vi "CHROMA Getting Started Main.vi"(8 "Error In":errorcluster) -> (0 "Error Out":errorcluster)   [LabVIEW 2016]
uses:
  Type Definition/CHROMA Voltage Range.ctl
  Type Definition/CHROMA Phase Shift Lines.ctl
  Type Definition/CHROMA Output State.ctl
  Type Definition/CHROMA Phase.ctl
panel:
  out "read buffer":string
  in  "Phase Shift Lines":T1
  in  "Phase Shift Angle":i32=180
  in  "Voltage Limit":i32=130
  in  "Voltage Range":T2=enum."Low (150V)"
  in  "Send":bool
  in  "Custom Command":string
  in  "Set 4":bool
  in  "Frequency":dbl=60.0 min=15.0 max=1200.0
  in  "Set 3":bool
  in  "Set 2":bool
  in  "Set 1":bool
  in  "Get System Status":bool
  out "Chroma Data":string[][](array[string])
  in  "Voltage Phase 3":dbl
  in  "Voltage Phase 2":dbl
  in  "Voltage Phase 1":dbl
  in  "Output Status":bool
  out "Instrument Name":string
  in  "Chroma VISA":refnum<visa-resource-name>="CHROMA"
  in  "Exit":bool
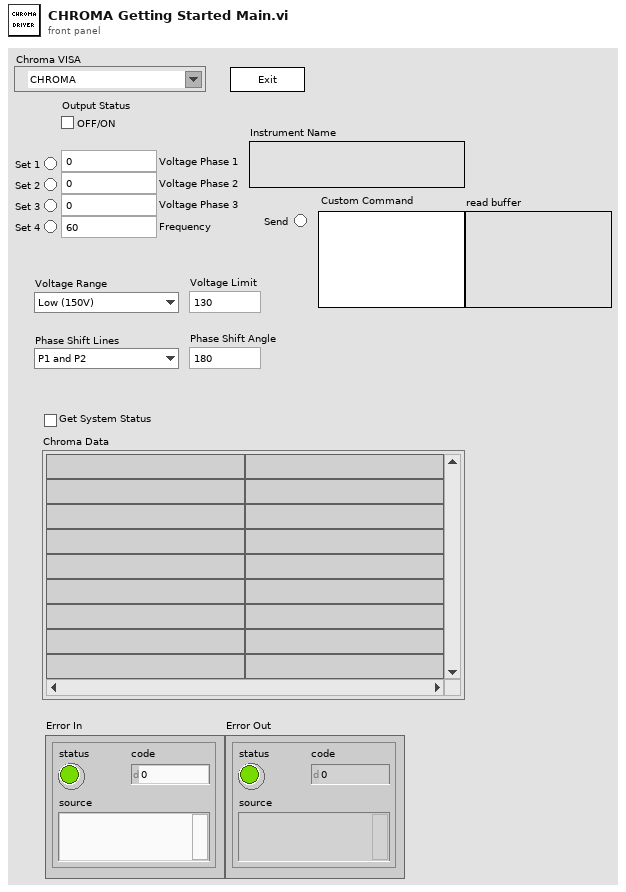
[diagram p1: front panel]
types:
  T1 = typedef "CHROMA Phase Shift Lines.ctl" = enum16{"P1 and P2", "P1 and P3"}
  T2 = typedef "CHROMA Voltage Range.ctl" = enum16{"High (300V)", "Low (150V)"}
  T3 = typedef "CHROMA Output State.ctl" = enum16{"Chroma OFF", "Chroma ON"}
  T4 = enum32{"invalid app kind", "Development System", "Run Time System", "Student Edition", "Embedded LabVIEW", "Evaluation", "Custom"}
  T5 = enum32{"Invalid", "Standard", "Closed", "Hidden", "Minimized", "Maximized"}
  T6 = typedef "CHROMA Phase.ctl" = enum16{"P1", "P2", "P3"}
  T7 = cluster{"Core":cluster{"Current VI Reference":refnum<vi>, "Close Panel on Exit?":bool}, "Chroma VISA":refnum<visa-resource-name>}
  T8 = cluster{"Current VI Reference":refnum<vi>, "Close Panel on Exit?":bool}
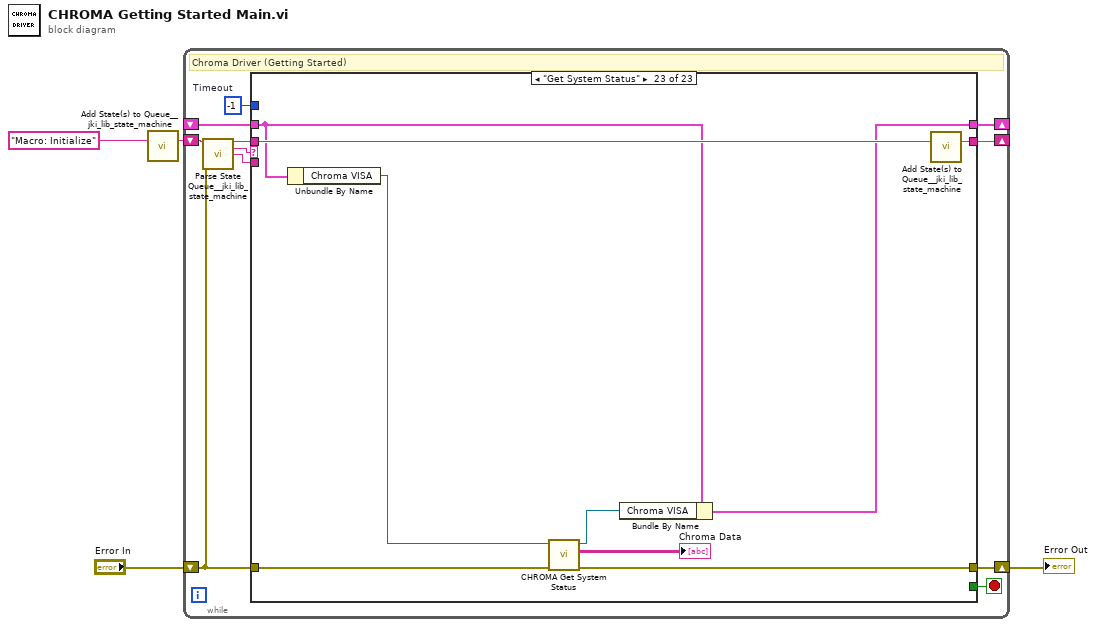
[diagram p0: block diagram]
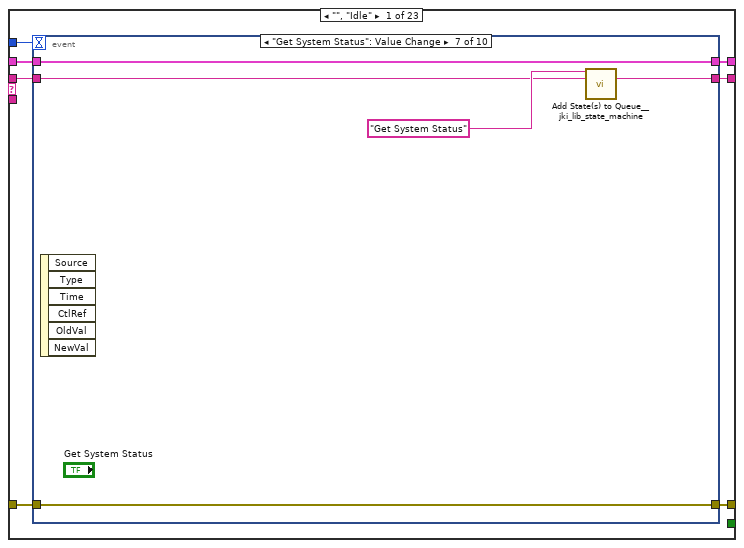
[diagram p2: hidden frame]
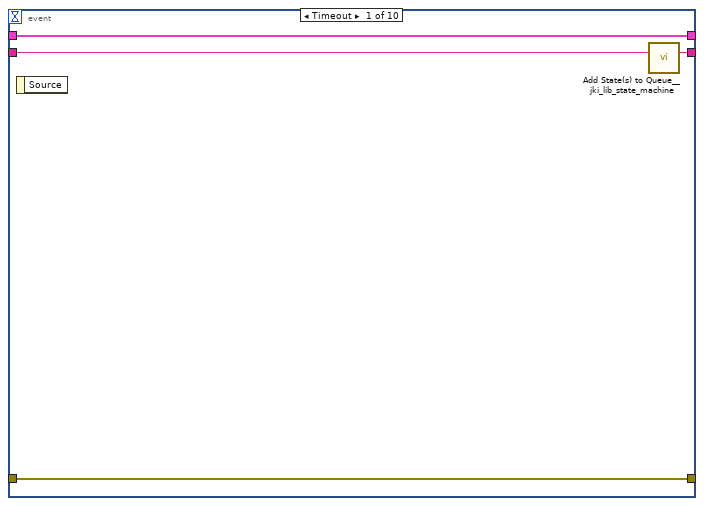
[diagram p3: hidden frame]
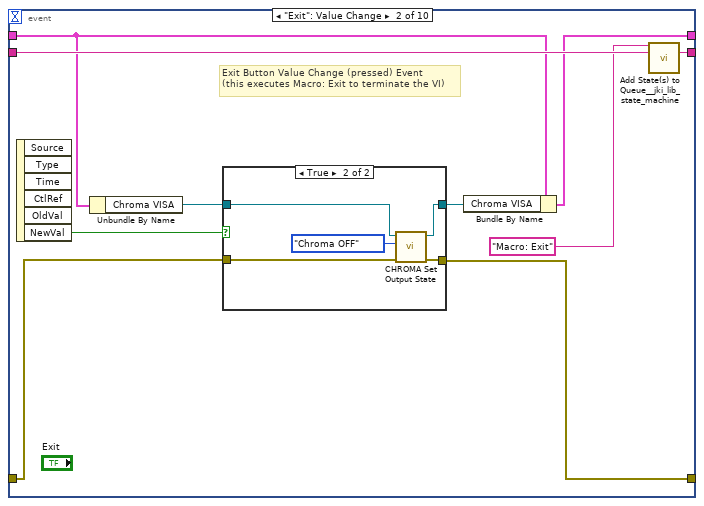
[diagram p4: hidden frame]
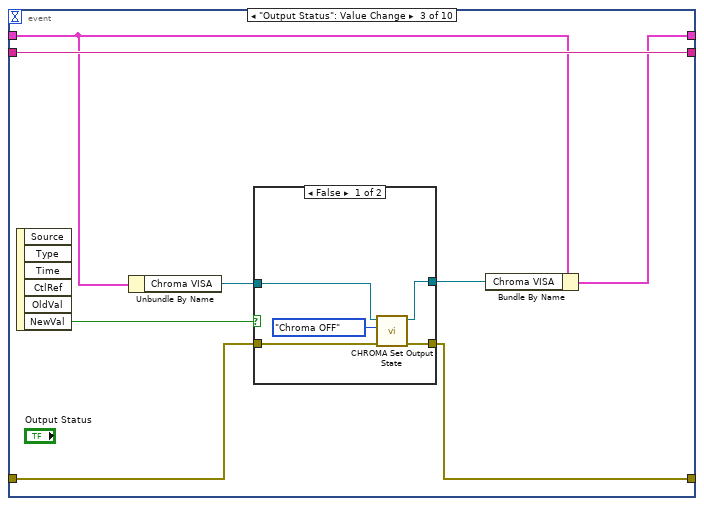
[diagram p6: hidden frame]
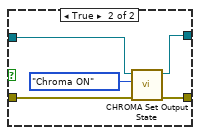
[diagram p7: hidden frame]
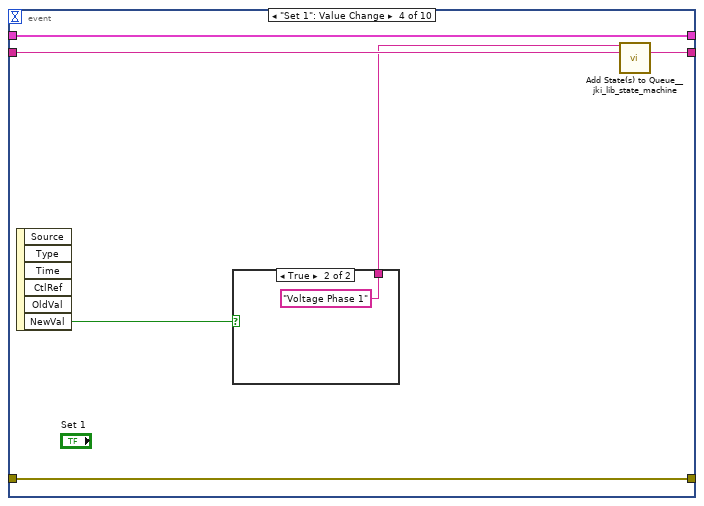
[diagram p8: hidden frame]
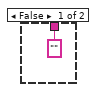
[diagram p9: hidden frame]
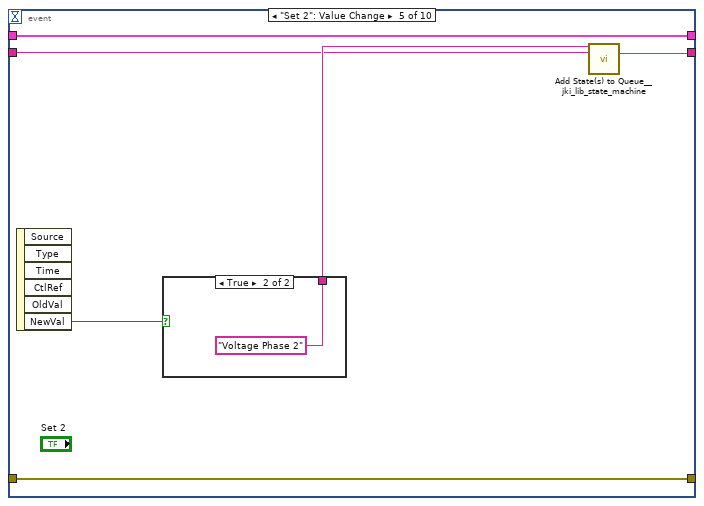
[diagram p10: hidden frame]
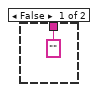
[diagram p11: hidden frame]
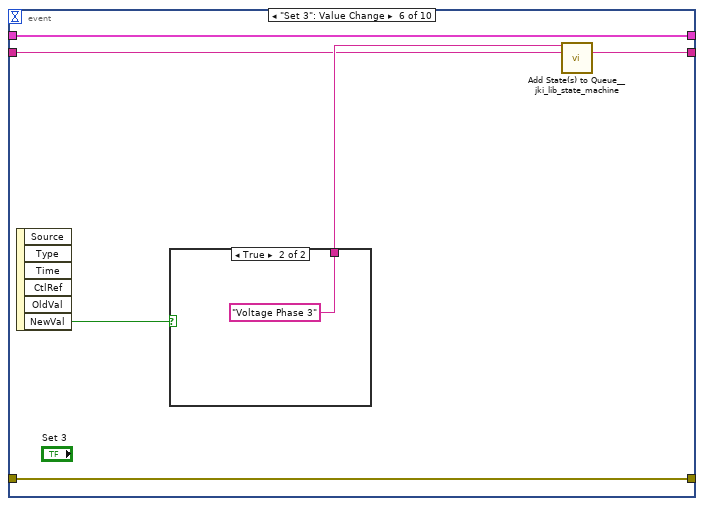
[diagram p12: hidden frame]
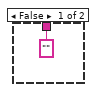
[diagram p13: hidden frame]
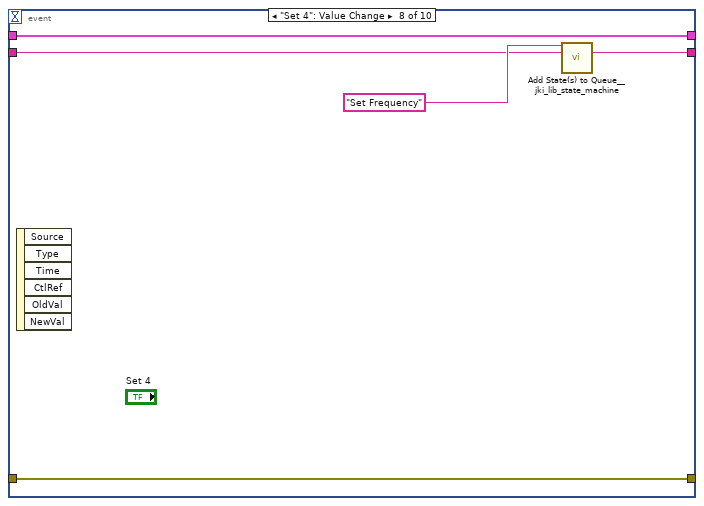
[diagram p14: hidden frame]
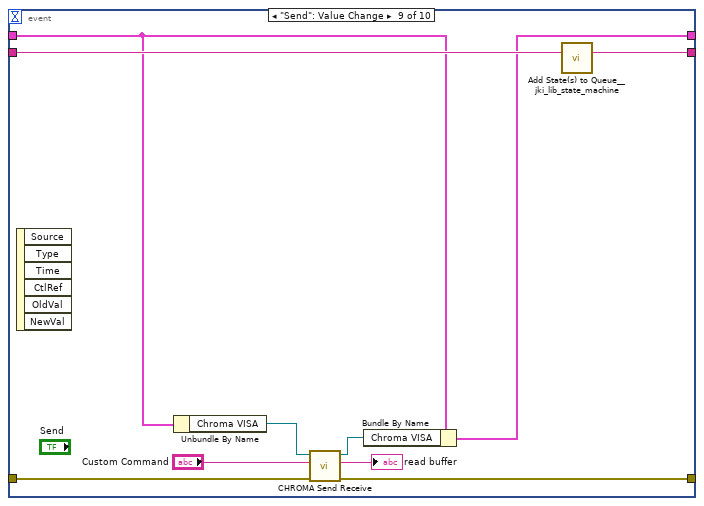
[diagram p15: hidden frame]
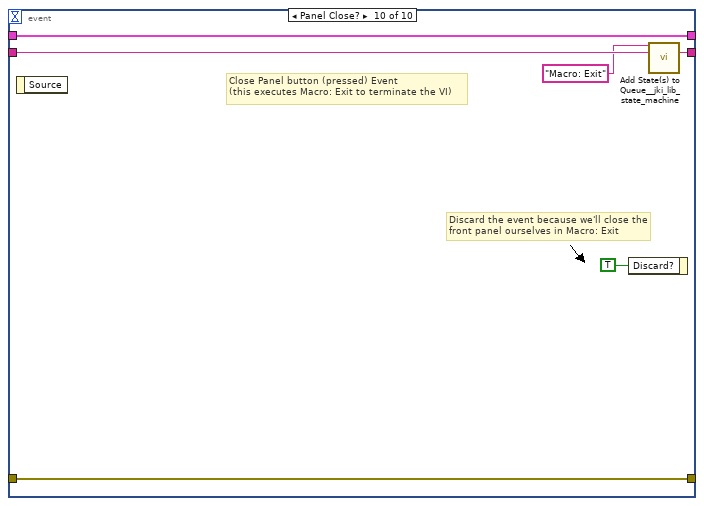
[diagram p16: hidden frame]
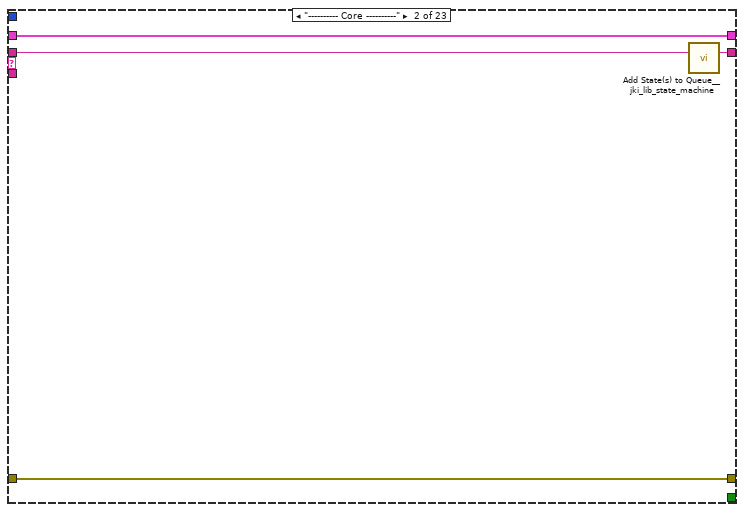
[diagram p17: hidden frame]
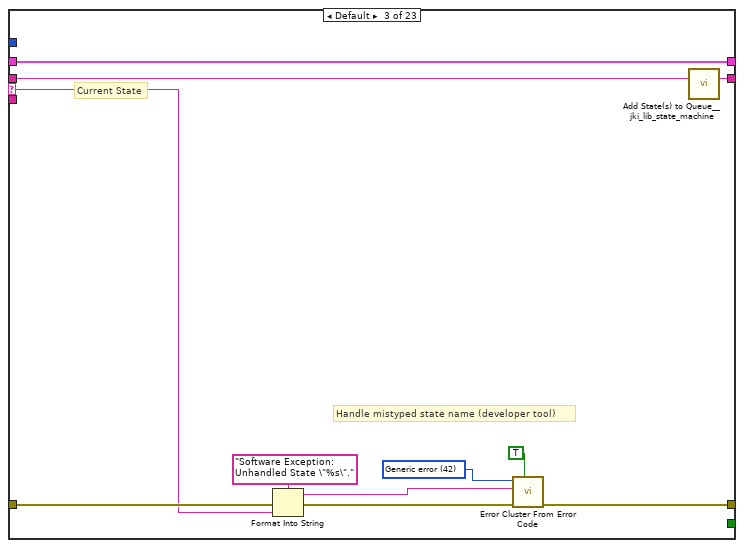
[diagram p18: hidden frame]
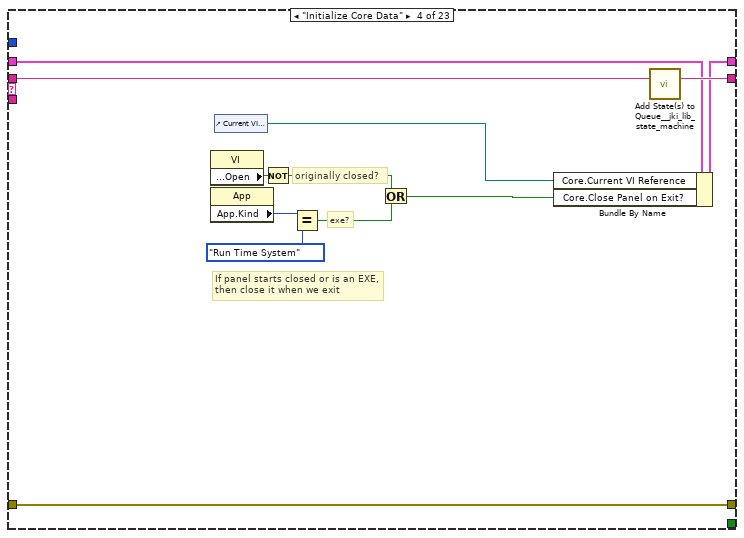
[diagram p19: hidden frame]
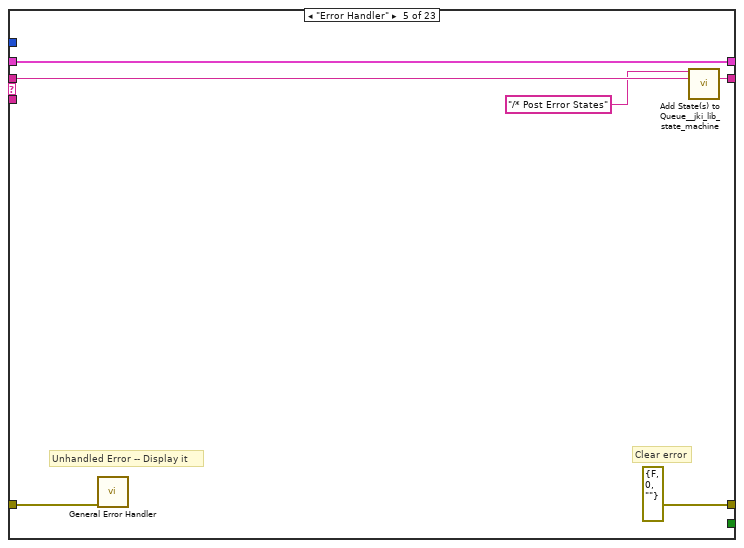
[diagram p20: hidden frame]
diagram:
  n1 = call <vilib>:"Add State(s) to Queue__jki_lib_state_machine.vi"("State(s) in (\"\")"="Macro: Initialize") -> ("States Out"=w4:string)  [unwired: 14 in]
  n2 = while "JKI - String-Based Queued State Machine (Basic) v1.0" {
    shift-right: [w8] -> _
    shift-left: _ -> [w7]
    shift-right: [w11] -> w2
    shift-left: "Error In" -> [w5]
    shift-right: [w10] -> _
    shift-left: w4 -> [w12]
    stop <- w9 stop-if-true
    w6 = -1  # Timeout
    # "Chroma Driver (Getting Started)"
    n3 = call <vilib>:"Parse State Queue__jki_lib_state_machine.vi"("State Queue"=w12, "Error In (no error)"=w5) -> ("Remaining States"=w14:string, "Current State"=w15:string, "Arguments"=w13:string)  [unwired: 11 in]
    n4 = case shown="\"Get System Status\"" w15 {
      selector: w15 -> [_ _ w116 _ _ _ _ _ _ _ _ _ _ _ _ _ _ _ _ _ _ _ _]
      tunnel: w14 -> [w22 w115 w120 w138 w144 w149 w153 w159 w171 w180 w184 w188 w194 w205 w231 w236 w246 w250 w260 w270 w280 w289 w298]
      tunnel: w13 -> [_ _ _ _ _ _ _ _ _ _ _ _ w189 w199 _ _ _ _ _ _ _ _ _]
      tunnel: w7 -> [w20 w112 w118 w129 w141 w147 w150 _ w166 w176 w181 w186 w192 w201 w228 w233 w243 w247 w253 w262 w273 w287 w292]
      tunnel: [w19 w113 w122 w135 errorcluster {"status"=FALSE, "code"=0, "source"=""} ("error out") w146 w151 w156 w168 w175 w182 w185 w190 w202 w229 w234 w244 w248 w257 w267 w277 w284 w295] -> w11
      tunnel: w5 -> [w18 w113 w121 w135 w140 w146 w151 w156 w169 w177 w182 w185 w191 w203 w229 w234 w244 w248 w258 w268 w278 w285 w296]
      tunnel: [w21 w114 w119 w137 w143 w148 w152 w158 w172 w179 w183 w187 w193 w204 w230 w235 w245 w249 w259 w269 w279 w288 w297] -> w10
      tunnel: [_ _ _ _ _ TRUE _ _ _ _ _ _ _ _ _ _ _ _ _ _ _ _ _] -> w9
      tunnel: [w17 w112 w118 w136 w141 w147 w150 w157 w165 w176 w181 w186 w192 w201 w228 w233 w243 w247 w252 w261 w272 w286 w291] -> w8
      tunnel: w6 -> [w16 _ _ _ _ _ _ _ _ _ _ _ _ _ _ _ _ _ _ _ _ _ _]
      frame "", "Idle" {
        n5 = event shown="[6] \"Get System Status\": Value Change" {
          selector: _ -> [_ _ _ _ _ _ _ _ _ _]
          dyn-events: _ -> [_ _ _ _ _ _ _ _ _ _]
          timeout: w16 -> [_ _ _ _ _ _ _ _ _ _]
          tunnel: w22 -> [w26 w36 w48 w65 w72 w81 w88 w93 w104 w111]
          tunnel: [w25 w35 w48 w66 w73 w82 w89 w94 w105 w110] -> w21
          tunnel: w20 -> [w23 w29 w46 w67 w75 w80 w87 w92 w98 w108]
          tunnel: [w24 w32 w49 w64 w71 w79 w86 w91 w102 w109] -> w19
          tunnel: w18 -> [w24 w33 w50 w64 w71 w79 w86 w91 w103 w109]
          tunnel: [w23 w28 w45 w67 w75 w80 w87 w92 w97 w108] -> w17
          event Timeout {
            n6 = event-data() -> ()  [unwired: 1 in, 1 out]
            n7 = call <vilib>:"Add State(s) to Queue__jki_lib_state_machine.vi"("State(s) in (\"\")"=w26) -> ("States Out"=w25:string)  [unwired: 14 in]
          }
          event "Exit": Value Change {
            # "Exit Button Value Change (pressed) Event\n(this executes Macro: Exit to terminate the VI)"
            n8 = event-data() -> ("NewVal"=w31:bool)  [unwired: 1 in, 5 out]
            n9 = Unbundle By Name(w29) -> ("Chroma VISA"=w30:refnum<visa-resource-name>)
            n10 = case shown="True" w31 {
              tunnel: w33 -> [w38 w42]
              tunnel: [w38 w41] -> w32
              tunnel: w30 -> [w37 w40]
              tunnel: [w37 w39] -> w27
              frame False {
              }
              frame True {
                n11 = call "CHROMA Set Output State.vi"("Error In"=w42, "Chroma Output State"=CHROMA_Output_State."Chroma OFF", "CHROMA VISA In"=w40) -> ("Error Out"=w41:errorcluster, "CHROMA VISA Out"=w39:refnum<visa-resource-name>)  [unwired: 6 in, 1 out]
              }
            }
            n12 = Bundle By Name(cluster=w29, "Chroma VISA"=w27) -> (w28:T7)
            n13 = call <vilib>:"Add State(s) to Queue__jki_lib_state_machine.vi"("State(s) in Front (\"\")"="Macro: Exit", "State(s) in (\"\")"=w36) -> ("States Out"=w35:string)  [unwired: 13 in]
          }
          event "Output Status": Value Change {
            n14 = event-data() -> ("NewVal"=w51:bool)  [unwired: 1 in, 5 out]
            n15 = Unbundle By Name(w46) -> ("Chroma VISA"=w47:refnum<visa-resource-name>)
            n16 = case shown="False" w51 {
              tunnel: w50 -> [w55 w60]
              tunnel: [w54 w59] -> w49
              tunnel: w47 -> [w53 w58]
              tunnel: [w52 w57] -> w44
              frame False {
                n17 = call "CHROMA Set Output State.vi"("Error In"=w55, "Chroma Output State"=CHROMA_Output_State."Chroma OFF", "CHROMA VISA In"=w53) -> ("Error Out"=w54:errorcluster, "CHROMA VISA Out"=w52:refnum<visa-resource-name>)  [unwired: 6 in, 1 out]
              }
              frame True {
                n18 = call "CHROMA Set Output State.vi"("Error In"=w60, "Chroma Output State"=CHROMA_Output_State."Chroma ON", "CHROMA VISA In"=w58) -> ("Error Out"=w59:errorcluster, "CHROMA VISA Out"=w57:refnum<visa-resource-name>)  [unwired: 6 in, 1 out]
              }
            }
            n19 = Bundle By Name(cluster=w46, "Chroma VISA"=w44) -> (w45:T7)
          }
          event "Set 1": Value Change {
            n20 = event-data() -> ("NewVal"=w62:bool)  [unwired: 1 in, 5 out]
            n21 = case shown="True" w62 {
              tunnel: ["" "Voltage Phase 1"] -> w63
              frame False {
              }
              frame True {
              }
            }
            n22 = call <vilib>:"Add State(s) to Queue__jki_lib_state_machine.vi"("State(s) in Front (\"\")"=w63, "State(s) in (\"\")"=w65) -> ("States Out"=w66:string)  [unwired: 13 in]
          }
          event "Set 2": Value Change {
            n23 = event-data() -> ("NewVal"=w70:bool)  [unwired: 1 in, 5 out]
            n24 = case shown="True" w70 {
              tunnel: ["" "Voltage Phase 2"] -> w74
              frame False {
              }
              frame True {
              }
            }
            n25 = call <vilib>:"Add State(s) to Queue__jki_lib_state_machine.vi"("State(s) in Front (\"\")"=w74, "State(s) in (\"\")"=w72) -> ("States Out"=w73:string)  [unwired: 13 in]
          }
          event "Set 3": Value Change {
            n26 = event-data() -> ("NewVal"=w78:bool)  [unwired: 1 in, 5 out]
            n27 = case shown="True" w78 {
              tunnel: ["" "Voltage Phase 3"] -> w83
              frame False {
              }
              frame True {
              }
            }
            n28 = call <vilib>:"Add State(s) to Queue__jki_lib_state_machine.vi"("State(s) in Front (\"\")"=w83, "State(s) in (\"\")"=w81) -> ("States Out"=w82:string)  [unwired: 13 in]
          }
          event "Get System Status": Value Change {
            n29 = event-data() -> ()  [unwired: 1 in, 6 out]
            n30 = call <vilib>:"Add State(s) to Queue__jki_lib_state_machine.vi"("State(s) in Front (\"\")"="Get System Status", "State(s) in (\"\")"=w88) -> ("States Out"=w89:string)  [unwired: 13 in]
          }
          event "Set 4": Value Change {
            n31 = event-data() -> ()  [unwired: 1 in, 6 out]
            n32 = call <vilib>:"Add State(s) to Queue__jki_lib_state_machine.vi"("State(s) in Front (\"\")"="Set Frequency", "State(s) in (\"\")"=w93) -> ("States Out"=w94:string)  [unwired: 13 in]
          }
          event "Send": Value Change {
            n33 = event-data() -> ()  [unwired: 1 in, 6 out]
            n34 = Unbundle By Name(w98) -> ("Chroma VISA"=w101:refnum<visa-resource-name>)
            n35 = call "CHROMA Send Receive.vi"("error in (no error)"=w103, "Send Command"="Custom Command", "CHROMA VISA In"=w101) -> ("error out"=w102:errorcluster, "read buffer"=→"read buffer":string, "CHROMA VISA Out"=w99:refnum<visa-resource-name>)  [unwired: 6 in]
            n36 = Bundle By Name(cluster=w98, "Chroma VISA"=w99) -> (w97:T7)
            n37 = call <vilib>:"Add State(s) to Queue__jki_lib_state_machine.vi"("State(s) in (\"\")"=w104) -> ("States Out"=w105:string)  [unwired: 14 in]
          }
          event Panel Close? {
            # "Discard the event because we'll close the front panel ourselves in Macro: Exit"
            # "Close Panel button (pressed) Event\n(this executes Macro: Exit to terminate the VI)"
            n38 = event-data() -> ()  [unwired: 1 in, 1 out]
            n39 = event-data("Discard?"=TRUE) -> ()  [unwired: 1 in, 1 out]
            n40 = call <vilib>:"Add State(s) to Queue__jki_lib_state_machine.vi"("State(s) in Front (\"\")"="Macro: Exit", "State(s) in (\"\")"=w111) -> ("States Out"=w110:string)  [unwired: 13 in]
          }
        }
      }
      frame "---------- Core ----------" {
        n41 = call <vilib>:"Add State(s) to Queue__jki_lib_state_machine.vi"("State(s) in (\"\")"=w115) -> ("States Out"=w114:string)  [unwired: 14 in]
      }
      frame Default {
        w125 = 42 items=["No error", "Argument error", "Memory is full", "Out of zone", "End of file", "File already open", "Generic file I/O error", "File not found", "File permission error", "Disk is full", "Duplicate path", "Too many files open", "System feature not enabled", "Resource file not found", "Cannot add resource", "Resource not found", "Image not found", "Image memory error", "Pen does not exist", "Config type invalid", "Config token not found", "Config parse error", "Config memory error", "Bad external code format", "Bad external code offset", "External code not present", "Null window", "Destroy window error", "Null menu", "Print aborted", "Bad print record", "Print driver error", "Windows error during printing", "Memory error during printing", "Print dialog error", "Generic print error", "Invalid device refnum", "Device not found", "Device parameter error", "Device unit error", "Cannot open device", "Device call aborted", "Generic error", "Cancelled by user", "Object ID too low", "Object ID too high", "Object not in heap", "Unknown heap", "Unknown object (invalid DefProc)", "Unknown object (DefProc not in table)", "Message out of range", "Invalid (null) method", "Unknown message", "Manager call not supported", "Bad address", "Network operation in progress", "Network operation timed out", "Connection is busy", "Network attribute not supported", "Network error", "Address in use", "System out of memory", "Connection aborted", "Connection refused", "Not connected", "Already connected", "Connection closed", "Initialization error (interapplication manager)", "Bad occurrence", "Wait on unbound occurrence handler", "Occurrence queue overflow", "Datalog type conflict", "Unused", "Unrecognized type (interapplication manager)", "Memory corrupt", "Failed to make temporary DLL", "Old CIN version", "Drag socket not found", "Failed to load drop-object", "Failed to register OLE object", "Failed to release OLE object", "Format specifier type mismatch", "Unknown format specifier", "Too few format specifiers", "Too many format specifiers", "Scan failed", "Newer CIN version", "Error converting to variant", "Runtime menu error", "Password tampered", "Variant attribute not found", "Incompatible variant data type", "Event data is not available", "Event Store is not present", "Occurrence is not found", "Event Queue is not created", "Event info is not available", "Refnum passed is NULL", "Error retrieving Class GUID", "Error retrieving CoClass GUID", "Error retrieving TypeLib GUID.", "Bad built application magic bytes.", "Specific driver is different from the specific driver associated with the Logical Name.", "There is no session opened to the class driver.", "Max Error", "MAX - Error with config objects", "MAX - Error loading configuration", "MAX - Group not supported"]
        # "Current State"
        # "Handle mistyped state name (developer tool)"
        n42 = Format Into String(format string="Software Exception: Unhandled State \"%s\"." ("message"), error in=w121, w116) -> (resulting string=w124:string, error out=w123:errorcluster)  [unwired: 1 in]
        n43 = call <vilib>:"Error Cluster From Error Code.vi"("show call chain? (False)"=TRUE, "error in (no error)"=w123, "error message (\"\")"=w124, "error code (0)"=w125) -> ("error out"=w122:errorcluster)  [unwired: 5 in]
        n44 = call <vilib>:"Add State(s) to Queue__jki_lib_state_machine.vi"("State(s) in (\"\")"=w120) -> ("States Out"=w119:string)  [unwired: 14 in]
      }
      frame "Initialize Core Data" {
        # "originally closed?"
        # "exe?"
        # "If panel starts closed or is an EXE, then close it when we exit"
        n45 = property class="VI"() -> ("Front Panel.Open"=w134:bool)  [unwired: 2 in, 2 out]
        n46 = property class="App"() -> ("App.Kind"=w133:T4)  [unwired: 2 in, 2 out]
        n47 = control-ref of="Current VI Reference"() -> (w127:refnum<vi>)
        n48 = Not(x=w134) -> (.not. x?=w131:bool)
        n49 = Equal?(x=w133, y=T4."Run Time System" ("Application:Kind")) -> (x = y?=w130:bool)
        n50 = Or(x=w131, y=w130) -> (x .or. y?=w128:bool)
        n51 = Bundle By Name(cluster=w129, "Core.Current VI Reference"=w127, "Core.Close Panel on Exit?"=w128) -> (w136:T7)
        n52 = call <vilib>:"Add State(s) to Queue__jki_lib_state_machine.vi"("State(s) in (\"\")"=w138) -> ("States Out"=w137:string)  [unwired: 14 in]
      }
      frame "Error Handler" {
        # "Unhandled Error -- Display it"
        # "Clear error"
        n53 = call <vilib>:"General Error Handler.vi"("error in (no error)"=w140) -> ()  [unwired: 10 in, 5 out]
        n54 = call <vilib>:"Add State(s) to Queue__jki_lib_state_machine.vi"("State(s) in Front (\"\")"="/* Post Error States", "State(s) in (\"\")"=w144) -> ("States Out"=w143:string)  [unwired: 13 in]
      }
      frame "Exit" {
        n55 = call <vilib>:"Add State(s) to Queue__jki_lib_state_machine.vi"("State(s) in (\"\")"=w149) -> ("States Out"=w148:string)  [unwired: 14 in]
      }
      frame "---------- Data ----------" {
        n56 = call <vilib>:"Add State(s) to Queue__jki_lib_state_machine.vi"("State(s) in (\"\")"=w153) -> ("States Out"=w152:string)  [unwired: 14 in]
      }
      frame "Data: Initialize" {
        w155 = T8 {"Current VI Reference"=refnum, "Close Panel on Exit?"=FALSE}  # Core
        n57 = Bundle("Core"=w155, "Chroma VISA"="Chroma VISA") -> (w157:T7)  [unwired: 1 in]
        n58 = call <vilib>:"Add State(s) to Queue__jki_lib_state_machine.vi"("State(s) in (\"\")"=w159) -> ("States Out"=w158:string)  [unwired: 14 in]
      }
      frame "Initialize Chroma" {
        n59 = Unbundle By Name(w166) -> ("Chroma VISA"=w170:refnum<visa-resource-name>)
        n60 = call "CHROMA Initialize.vi"("Phase Shift Lines"="Phase Shift Lines", "Phase Shift Angle"="Phase Shift Angle", "Error In"=w169, "Voltage Limit"="Voltage Limit", "Voltage Range"="Voltage Range", "CHROMA VISA In"=w170) -> ("Error Out"=w168:errorcluster, "Instrument Name"=→"Instrument Name":string, "CHROMA VISA Out"=w164:refnum<visa-resource-name>)  [unwired: 3 in]
        n61 = Bundle By Name(cluster=w166, "Chroma VISA"=w164) -> (w165:T7)
        n62 = call <vilib>:"Add State(s) to Queue__jki_lib_state_machine.vi"("State(s) in (\"\")"=w171) -> ("States Out"=w172:string)  [unwired: 14 in]
      }
      frame "Data: Cleanup" {
        n63 = Unbundle By Name(w176) -> ("Chroma VISA"=w174:refnum<visa-resource-name>, "Core.Current VI Reference"=w178:refnum<vi>)
        n64 = Close Reference(reference=w178, error in (no error)=w177) -> (error out=w173:errorcluster)
        n65 = VISA Close(VISA resource name=w174, error in (no error)=w173) -> (error out=w175:errorcluster)
        n66 = call <vilib>:"Add State(s) to Queue__jki_lib_state_machine.vi"("State(s) in (\"\")"=w180) -> ("States Out"=w179:string)  [unwired: 14 in]
      }
      frame "---------- UI ----------" {
        n67 = call <vilib>:"Add State(s) to Queue__jki_lib_state_machine.vi"("State(s) in (\"\")"=w184) -> ("States Out"=w183:string)  [unwired: 14 in]
      }
      frame "UI: Initialize" {
        n68 = call <vilib>:"Add State(s) to Queue__jki_lib_state_machine.vi"("State(s) in (\"\")"=w188) -> ("States Out"=w187:string)  [unwired: 14 in]
      }
      frame "UI: Cursor Set" {
        # "Argument"
        n69 = case shown="\"Idle\", Default" w189 {
          tunnel: w191 -> [w196 w198]
          tunnel: [w195 w197] -> w190
          frame "Idle", Default {
            n70 = call <vilib>:"Unset Busy.vi"("error in (no error)"=w196) -> ("error out"=w195:errorcluster)  [unwired: 10 in]
          }
          frame "Busy" {
            n71 = call <vilib>:"Set Busy.vi"("error in (no error)"=w198) -> ("error out"=w197:errorcluster)  [unwired: 9 in, 1 out]
          }
        }
        n72 = call <vilib>:"Add State(s) to Queue__jki_lib_state_machine.vi"("State(s) in (\"\")"=w194) -> ("States Out"=w193:string)  [unwired: 14 in]
      }
      frame "UI: Front Panel State" {
        # "Argument"
        n73 = Unbundle By Name(w201) -> ("Core.Current VI Reference"=w200:refnum<vi>)
        n74 = case shown="\"Open\", Default" w199 {
          tunnel: w203 -> [w209 w222]
          tunnel: [w211 w223] -> w202
          tunnel: w200 -> [w210 w220]
          frame "Open", Default {
            n75 = property class="VI"(reference=w210, error in=w209) -> (reference out=w207:refnum<vi>, error out=w208:errorcluster, "Front Panel.Open"=w206:bool)
            n76 = case shown="False" w206 {
              tunnel: [w214 w217] -> w211
              tunnel: w208 -> [w213 w217]
              tunnel: w207 -> [w212 _]
              frame False {
                n77 = invoke class="VI" method="FP.Open"(reference=w212, error in=w213, "Activate"=TRUE, "State"=T5."Standard") -> (error out=w214:errorcluster)  [unwired: 1 in, 4 out]
              }
              frame True {
              }
            }
          }
          frame "Close" {
            n78 = property class="VI"(reference=w220, error in=w222) -> (reference out=w219:refnum<vi>, error out=w221:errorcluster, "Front Panel.Open"=w218:bool)
            n79 = case shown="True" w218 {
              tunnel: [w224 w227] -> w223
              tunnel: w221 -> [w224 w226]
              tunnel: w219 -> [_ w225]
              frame False {
              }
              frame True {
                n80 = invoke class="VI" method="FP.Close"(reference=w225, error in=w226) -> (error out=w227:errorcluster)  [unwired: 1 in, 2 out]
              }
            }
          }
        }
        n81 = call <vilib>:"Add State(s) to Queue__jki_lib_state_machine.vi"("State(s) in (\"\")"=w205) -> ("States Out"=w204:string)  [unwired: 14 in]
      }
      frame "---------- Macro ----------" {
        n82 = call <vilib>:"Add State(s) to Queue__jki_lib_state_machine.vi"("State(s) in (\"\")"=w231) -> ("States Out"=w230:string)  [unwired: 14 in]
      }
      frame "Macro: Initialize" {
        w232 = "Data: Initialize\nInitialize Core Data\nUI: Initialize\nUI: Front Panel State >> Open\nInitialize Chroma"  # Data: Initialize Initialize Core Data UI: Initialize UI: Front Panel State >> Open Initialize Chroma
        n83 = call <vilib>:"Add State(s) to Queue__jki_lib_state_machine.vi"("State(s) in Front (\"\")"=w232, "State(s) in (\"\")"=w236) -> ("States Out"=w235:string)  [unwired: 13 in]
      }
      frame "Macro: Exit" {
        n84 = Unbundle By Name(w243) -> ("Core.Close Panel on Exit?"=w242:bool)
        n85 = Select(t="UI: Front Panel State >> Close", s=w242, f="") -> (s? t:f=w239:string)
        n86 = call <vilib>:"Add State(s) to Queue__jki_lib_state_machine.vi"("State(s) in (\"\")"=w239, "State(s) at Back (\"\")"="Data: Cleanup\nExit") -> ("States Out"=w237:string)  [unwired: 13 in]
        n87 = call <vilib>:"Add State(s) to Queue__jki_lib_state_machine.vi"("State(s) in Front (\"\")"=w237, "State(s) in (\"\")"=w246) -> ("States Out"=w245:string)  [unwired: 13 in]
      }
      frame "---------- New Category ----------" {
        n88 = call <vilib>:"Add State(s) to Queue__jki_lib_state_machine.vi"("State(s) in (\"\")"=w250) -> ("States Out"=w249:string)  [unwired: 14 in]
      }
      frame "Voltage Phase 1" {
        n89 = Unbundle By Name(w253) -> ("Chroma VISA"=w255:refnum<visa-resource-name>)
        n90 = call "CHROMA Set Voltage.vi"("Phase"=CHROMA_Phase."P1", "Error In"=w258, "Voltage Setpoint"="Voltage Phase 1", "CHROMA VISA In"=w255) -> ("Error Out"=w257:errorcluster, "CHROMA VISA Out"=w251:refnum<visa-resource-name>)  [unwired: 6 in]
        n91 = Bundle By Name(cluster=w253, "Chroma VISA"=w251) -> (w252:T7)
        n92 = call <vilib>:"Add State(s) to Queue__jki_lib_state_machine.vi"("State(s) in (\"\")"=w260) -> ("States Out"=w259:string)  [unwired: 14 in]
      }
      frame "Voltage Phase 2" {
        n93 = Unbundle By Name(w262) -> ("Chroma VISA"=w265:refnum<visa-resource-name>)
        n94 = call "CHROMA Set Voltage.vi"("Phase"=CHROMA_Phase."P2", "Error In"=w268, "Voltage Setpoint"="Voltage Phase 2", "CHROMA VISA In"=w265) -> ("Error Out"=w267:errorcluster, "CHROMA VISA Out"=w263:refnum<visa-resource-name>)  [unwired: 6 in]
        n95 = Bundle By Name(cluster=w262, "Chroma VISA"=w263) -> (w261:T7)
        n96 = call <vilib>:"Add State(s) to Queue__jki_lib_state_machine.vi"("State(s) in (\"\")"=w270) -> ("States Out"=w269:string)  [unwired: 14 in]
      }
      frame "Voltage Phase 3" {
        n97 = Unbundle By Name(w273) -> ("Chroma VISA"=w276:refnum<visa-resource-name>)
        n98 = call "CHROMA Set Voltage.vi"("Phase"=CHROMA_Phase."P3", "Error In"=w278, "Voltage Setpoint"="Voltage Phase 3", "CHROMA VISA In"=w276) -> ("Error Out"=w277:errorcluster, "CHROMA VISA Out"=w271:refnum<visa-resource-name>)  [unwired: 6 in]
        n99 = Bundle By Name(cluster=w273, "Chroma VISA"=w271) -> (w272:T7)
        n100 = call <vilib>:"Add State(s) to Queue__jki_lib_state_machine.vi"("State(s) in (\"\")"=w280) -> ("States Out"=w279:string)  [unwired: 14 in]
      }
      frame "Set Frequency" {
        n101 = Unbundle By Name(w287) -> ("Chroma VISA"=w282:refnum<visa-resource-name>)
        n102 = call "CHROMA Set Frequency.vi"("Error In"=w285, "Frequency"="Frequency", "CHROMA VISA In"=w282) -> ("Error Out"=w284:errorcluster, "CHROMA VISA Out"=w283:refnum<visa-resource-name>)  [unwired: 7 in]
        n103 = Bundle By Name(cluster=w287, "Chroma VISA"=w283) -> (w286:T7)
        n104 = call <vilib>:"Add State(s) to Queue__jki_lib_state_machine.vi"("State(s) in (\"\")"=w289) -> ("States Out"=w288:string)  [unwired: 14 in]
      }
      frame "Get System Status" {
        n105 = Unbundle By Name(w292) -> ("Chroma VISA"=w294:refnum<visa-resource-name>)
        n106 = call "CHROMA Get System Status.vi"("Error In"=w296, "CHROMA VISA In"=w294) -> ("Error Out"=w295:errorcluster, "Chroma Data"=→"Chroma Data":string[][], "CHROMA VISA Out"=w290:refnum<visa-resource-name>)  [unwired: 7 in]
        n107 = Bundle By Name(cluster=w292, "Chroma VISA"=w290) -> (w291:T7)
        n108 = call <vilib>:"Add State(s) to Queue__jki_lib_state_machine.vi"("State(s) in (\"\")"=w298) -> ("States Out"=w297:string)  [unwired: 14 in]
      }
    }
  }
  "Error Out" <- w2
